vi "Team Map.vi"(11 "Map in":refnum<class "Map.lvclass">) -> (2 "Team Map":i32[][](array[numeric]), 3 "Map out":refnum<class "Map.lvclass">)   [LabVIEW 2020, in "SquareBattle.lvlib" / "Map.lvclass"]
uses:
  Map.lvclass
  Map.lvclass/Map.ctl
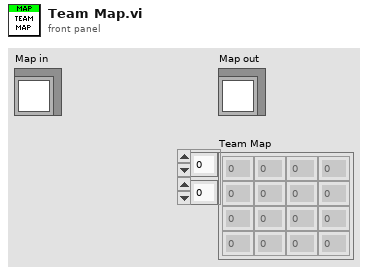
[diagram p1: front panel]
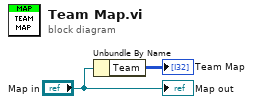
[diagram p0: block diagram]
diagram:
  n1 = Unbundle By Name("Map in") -> ("Team"=→"Team Map":i32[][])
  "Map out" <- "Map in"
